vi "Rohde & Schwarz VNA Set Power.vi"(6 "Channel":i8=1 min=1 max=99 step=1, 7 "Rohde & Schwarz VNA":T1, 8 "error in (no error)":errorcluster, 10 "Source Power, dBm (0.0)":dbl, 11 "VISA Resource Name":refnum<visa-resource-name>) -> (0 "error out":errorcluster, 3 "dup VISA Resource Name":refnum<visa-resource-name>)   [LabVIEW 2011]
doc: "This vi sets the power range. Only works on the HP 8753D."
uses:
  TypeDefs/Rohde & Schwarz VNA Instrument Info.ctl
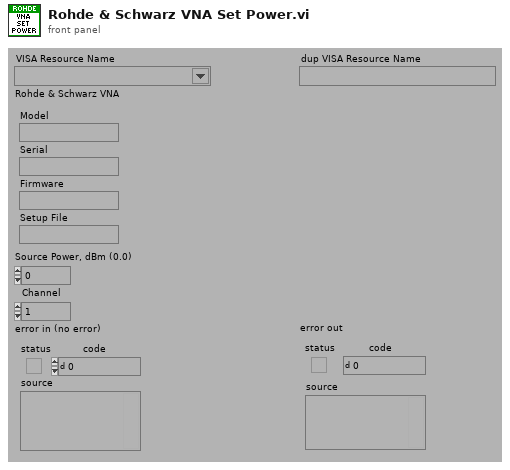
[diagram p1: front panel]
types:
  T1 = typedef "Rohde & Schwarz VNA Instrument Info.ctl" = cluster{"Model":string, "Serial":string, "Firmware":string, "Setup File":string}
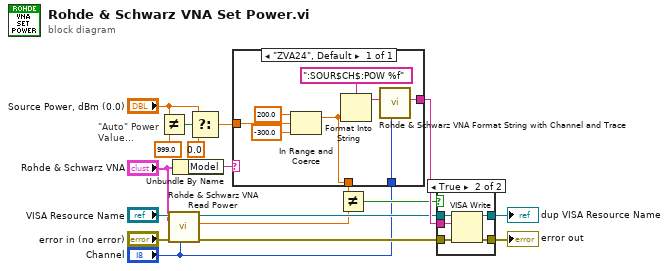
[diagram p0: block diagram]
diagram:
  # "\"Auto\" Power\nValue..."
  n1 = Not Equal?(x="Source Power, dBm (0.0)", y=999.0) -> (x != y?=w6:bool)
  n2 = call "Rohde & Schwarz VNA Read Power.vi"("Channel"="Channel", "Rohde & Schwarz VNA"="Rohde & Schwarz VNA", "error in (no error)"="error in (no error)", "VISA Resource Name"="VISA Resource Name") -> ("error out"=w13:errorcluster, "Source Power, dBm"=w10:dbl, "dup VISA Resource Name"=w11:refnum<visa-resource-name>)  [unwired: 5 out]
  n3 = Unbundle By Name("Rohde & Schwarz VNA") -> ("Model"=w1:string)
  n4 = Select(t="Source Power, dBm (0.0)", s=w6, f=0.0) -> (s? t:f=w4:dbl)
  n5 = case shown="\"ZVA24\", Default" w1 {
    tunnel: [w20] -> w15
    tunnel: w4 -> [w23]
    tunnel: [w22] -> w8
    tunnel: "Channel" -> [w19]
    frame "ZVA24", Default {
      n6 = In Range and Coerce(upper limit=200.0, x=w23, lower limit=-300.0) -> (coerced(x)=w22:dbl)  [unwired: 1 out]
      n7 = Format Into String(format string=":SOUR$CH$:POW %f", w22) -> (resulting string=w21:string)  [unwired: 2 in, 1 out]
      n8 = call "Rohde & Schwarz VNA Format String with Channel and Trace.vi"("Channel"=w19, "String"=w21) -> ("String Out"=w20:string)  [unwired: 1 in, 6 out]
    }
  }
  n9 = Not Equal?(x=w8, y=w10) -> (x != y?=w9:bool)
  n10 = case shown="True" w9 {
    tunnel: [w27 w33] -> w18
    tunnel: [w28 w32] -> w17
    tunnel: w15 -> [_ w31]
    tunnel: w13 -> [w27 w30]
    tunnel: w11 -> [w28 w29]
    frame False {
    }
    frame True {
      n11 = VISA Write(VISA resource name=w29, write buffer=w31, error in (no error)=w30) -> (VISA resource name out=w32:refnum<visa-resource-name>, error out=w33:errorcluster)  [unwired: 1 out]
    }
  }
  "dup VISA Resource Name" <- w17
  "error out" <- w18
